vi "start.vi"(8 "error in (no error)":errorcluster, 11 "DDSOutput in":refnum<class "DDSOutput.lvclass">) -> (0 "error out":errorcluster, 3 "DDSOutput out":refnum<class "DDSOutput.lvclass">)   [LabVIEW 2011, in "Hardware.lvlib" / "Channels.lvlib" / "DDSOutput.lvclass"]
uses:
  DDSOutput.lvclass
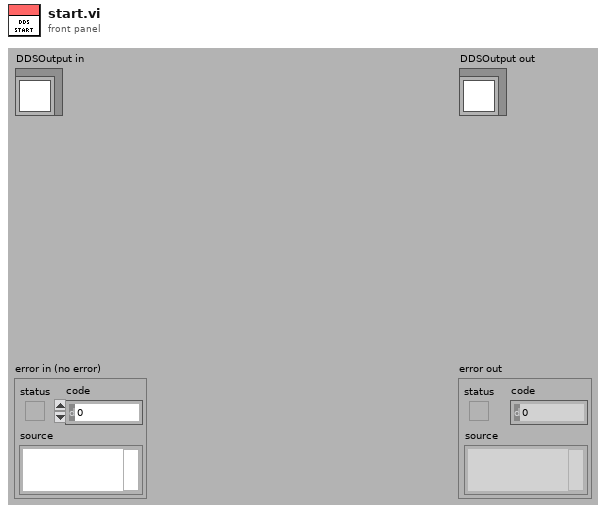
[diagram p1: front panel]
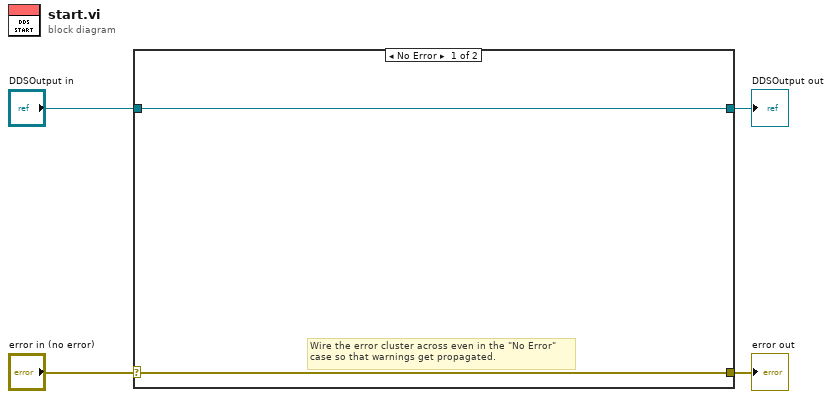
[diagram p0: block diagram]
diagram:
  n1 = case shown="No Error" "error in (no error)" {
    selector: "error in (no error)" -> [w5 w8]
    tunnel: [w5 w8] -> w3
    tunnel: [w6 w7] -> w1
    tunnel: "DDSOutput in" -> [w6 w7]
    frame No Error {
      # "Wire the error cluster across even in the \"No Error\"\ncase so that warnings get propagated."
    }
    frame Error {
    }
  }
  "error out" <- w3
  "DDSOutput out" <- w1
